vi "ATM_account_handler.vi"(7 "Action":enum16{"Read User Info", "Update User Info"}(ring), 9 "Users info (for update)":string[](array[string]), 10 "User Input (for read)":string) -> (2 "Users info":string[](array[string]))   [LabVIEW 2025]
doc: "This VI handles the “ATM accounts.txt” file.\nIf the Action is set to “Read User Info”, it will return in a four elements 1D string ARRAY the informations of this account. If the account doesn’t exists, it will return an empty four elements 1D string ARRAY.\nIf the Action is set to “Update User Info”, it will update the “ATM accounts.txt” file with the informations given in the Users info (for update) control"
uses:
  <vilib>/Utility/file.llb/Read Delimited Spreadsheet (string).vi
  <vilib>/Utility/file.llb/Write Delimited Spreadsheet (string).vi
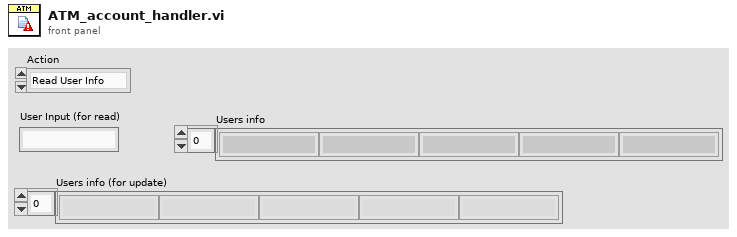
[diagram p1: front panel]
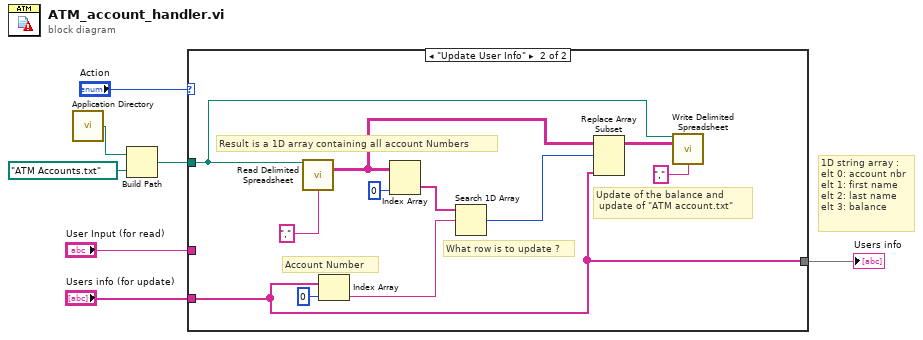
[diagram p0: block diagram]
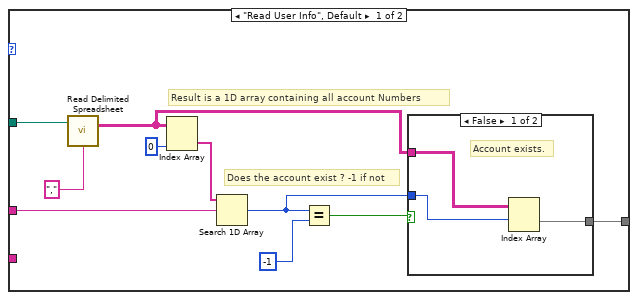
[diagram p2: hidden frame]
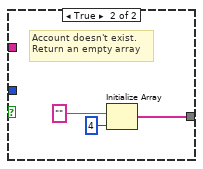
[diagram p3: hidden frame]
diagram:
  # "1D string array :\nelt 0: account nbr\nelt 1: first name\nelt 2: last name\nelt 3: balance"
  n1 = call <vilib>:"Application Directory.vi"() -> ("Application Directory"=w5:path)
  n2 = Build Path(base path=w5, name or relative path=path "ATM Accounts.txt") -> (appended path=w4:path)
  n3 = case shown="\"Update User Info\"" "Action" {
    tunnel: w4 -> [w17 w26]
    tunnel: "User Input (for read)" -> [w13 _]
    tunnel: [w10 w24] -> w2
    tunnel: "Users info (for update)" -> [_ w24]
    frame "Read User Info", Default {
      # "Does the account exist ? -1 if not"
      # "Result is a 1D array containing all account Numbers"
      n4 = call-poly <vilib>:"Read Delimited Spreadsheet.vi"("file path (dialog if empty)"=w17, "delimiter (\\t)"="," ("delimiter (\\t)")) -> ("all rows"=w9:string[][])  [unwired: 8 in, 5 out]
      n5 = Index Array(array=w9, index (col)=0 ("disabled index (col)")) -> (element=w14:string[])  [unwired: 1 in]
      n6 = Search 1D Array(1D array=w14, element=w13) -> (index of element=w8:i32)  [unwired: 1 in]
      n7 = Equal?(x=w8, y=-1) -> (x = y?=w11:bool)
      n8 = case shown="False" w11 {
        tunnel: [w18 w21] -> w10
        tunnel: w9 -> [w20 _]
        tunnel: w8 -> [w19 _]
        frame False {
          # "Account exists."
          n9 = Index Array(array=w20, index (row)=w19) -> (element=w18:string[])  [unwired: 1 in]
        }
        frame True {
          # "Account doesn't exist.\nReturn an empty array"
          n10 = Initialize Array("", 4 ("dimension size")) -> (w21:string[])
        }
      }
    }
    frame "Update User Info" {
      # "Update of the balance and\n update of \"ATM account.txt\""
      # "What row is to update ?"
      # "Account Number"
      # "Result is a 1D array containing all account Numbers"
      n11 = call-poly <vilib>:"Read Delimited Spreadsheet.vi"("file path (dialog if empty)"=w26, "delimiter (\\t)"="," ("delimiter (\\t)")) -> ("all rows"=w29:string[][])  [unwired: 8 in, 5 out]
      n12 = Index Array(array=w24, index=0) -> (element=w30:string)
      n13 = Index Array(array=w29, index (col)=0 ("disabled index (col)")) -> (element=w31:string[])  [unwired: 1 in]
      n14 = Search 1D Array(1D array=w31, element=w30) -> (index of element=w28:i32)  [unwired: 1 in]
      n15 = Replace Array Subset(array=w29, new element=w24, index (row)=w28) -> (w27:string[][])  [unwired: 1 in]
      n16 = call-poly <vilib>:"Write Delimited Spreadsheet.vi"("file path (dialog if empty)"=w26, "2D data"=w27, "delimiter (\\t)"="," ("delimiter (\\t)")) -> ()  [unwired: 11 in, 2 out]
    }
  }
  "Users info" <- w2
